vi "LVIS_FileSize.vi"(8 "Error In":errorcluster, 11 "State In":bool) -> (0 "Error out":errorcluster, 3 "State Out":bool)   [LabVIEW 2015]
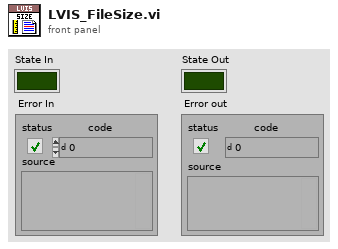
[diagram p1: front panel]
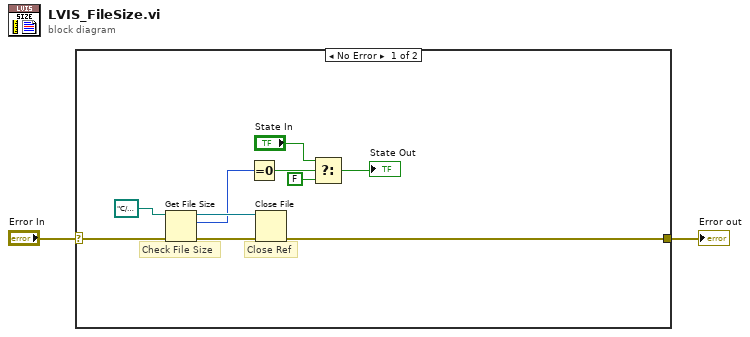
[diagram p0: block diagram]
diagram:
  n1 = case shown="No Error" "Error In" {
    selector: "Error In" -> [w12 w13]
    tunnel: [w7 w13] -> w1
    frame No Error {
      # "Close Ref"
      # "Check File Size"
      n2 = Get File Size(file=path "C:/Medtronic/Labview/LVIS Library/LVIS_Settings.ini" ("file path (use dialog)"), error in=w12) -> (refnum out=w9:refnum<file>, size (in bytes)=w8:i64, 0:w10:errorcluster)
      n3 = Equal To 0?(x=w8) -> (x = 0?=w6:bool)
      n4 = Close File(refnum=w9, error in=w10) -> (error out=w7:errorcluster)  [unwired: 1 out]
      n5 = Select(t="State In", s=w6, f=FALSE) -> (s? t:f=→"State Out":bool)
    }
    frame Error {
    }
  }
  "Error out" <- w1
